vi "WriteName.vi"(8 "error in (no error)":errorcluster, 10 "Name":string, 11 "Step in":refnum<class "Step.lvclass">) -> (0 "error out":errorcluster, 3 "Step out":refnum<class "Step.lvclass">)   [LabVIEW 2023, in "Easy.SequenceManagerLabVIEW.lvlib" / "Step.lvclass"]
uses:
  Step.lvclass
  Step.lvclass/Step.ctl
panel:
  # "Connector Pane"
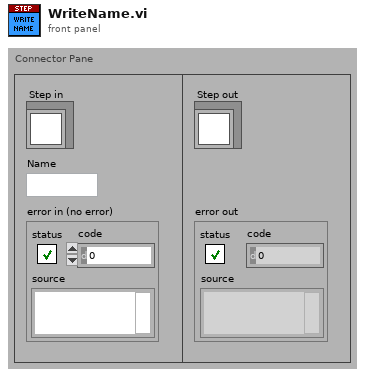
[diagram p1: front panel]
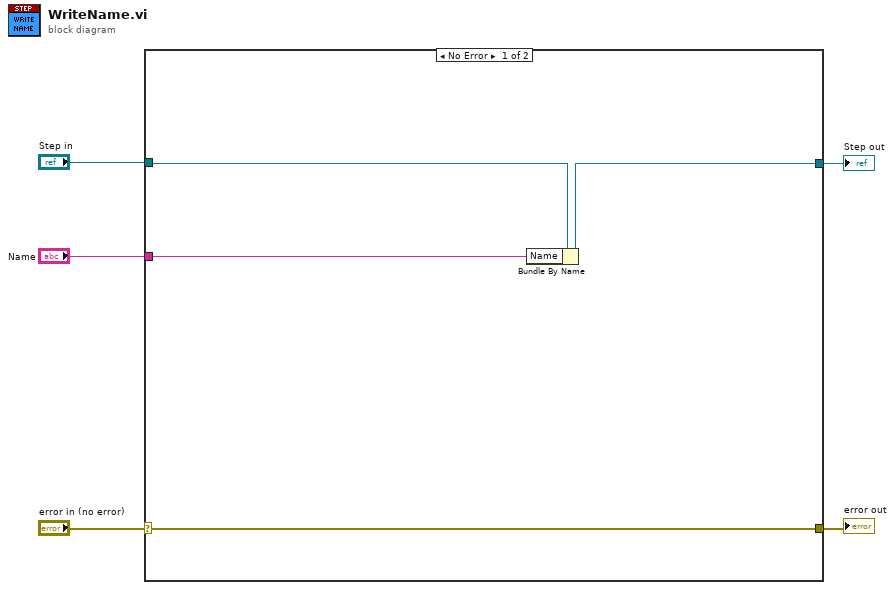
[diagram p0: block diagram]
diagram:
  n1 = case shown="No Error" "error in (no error)" {
    selector: "error in (no error)" -> [w8 w11]
    tunnel: [w8 w11] -> w4
    tunnel: [w6 w10] -> w2
    tunnel: "Step in" -> [w7 w10]
    tunnel: "Name" -> [w9 _]
    frame No Error {
      n2 = Bundle By Name(cluster=w7, "Name"=w9) -> (w6:refnum<class "Step.lvclass">)
    }
    frame Error {
    }
  }
  "error out" <- w4
  "Step out" <- w2
